vi "Get Common Image Resolution.vi"(11 "Array of Image Resolutions":T1(array[cluster])) -> (1 "Single Resolution":bool, 2 "Y Resolution":i32, 3 "X Resolution":i32)   [LabVIEW 2021, in "Image.lvlib"]
uses:
  d99703d1-a6cb-43ff-b6d2-b2996db2618f.vi
  72ccfe63-be56-4aee-b994-c4e655807a49.vi
  Image.lvlib
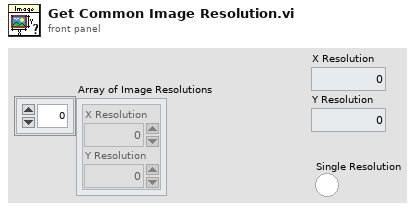
[diagram p1: front panel]
types:
  T1 = cluster{"X Resolution":i32, "Y Resolution":i32}[]
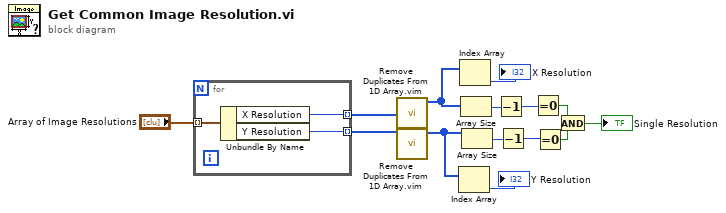
[diagram p0: block diagram]
diagram:
  n1 = for {
    tunnel: "Array of Image Resolutions" -> [w17] mode=indexing
    tunnel: [w16] -> w13 mode=indexing
    tunnel: [w15] -> w12 mode=indexing
    n2 = Unbundle By Name(w17) -> ("X Resolution"=w16:i32, "Y Resolution"=w15:i32)
  }
  n3 = call "Remove Duplicates From 1D Array.vim"("array"=w13) -> ("array with duplicates removed"=w7:i32[])  [unwired: 10 in]
  n4 = call "Remove Duplicates From 1D Array.vim"("array"=w12) -> ("array with duplicates removed"=w6:i32[])  [unwired: 10 in]
  n5 = Index Array(array=w6) -> (element=→"Y Resolution":i32)  [unwired: 1 in]
  n6 = Index Array(array=w7) -> (element=→"X Resolution":i32)  [unwired: 1 in]
  n7 = Array Size(array=w7) -> (size(s)=w11:i32)
  n8 = Array Size(array=w6) -> (size(s)=w10:i32)
  n9 = Decrement(x=w11) -> (x-1=w9:i32)
  n10 = Decrement(x=w10) -> (x-1=w8:i32)
  n11 = Equal To 0?(x=w9) -> (x = 0?=w3:bool)
  n12 = Equal To 0?(x=w8) -> (x = 0?=w2:bool)
  n13 = And(x=w3, y=w2) -> (x .and. y?=→"Single Resolution":bool)
